vi "plot_side_cutting_offset.vi"(10 "index":dbl, 11 "coord cluster":cluster{dbl[][]}[](array[cluster])) -> (2 "End Point out":cluster{"X":i32, "Y":i32}, 3 "Start Point out":cluster{"X":i32, "Y":i32})   [LabVIEW 2017]
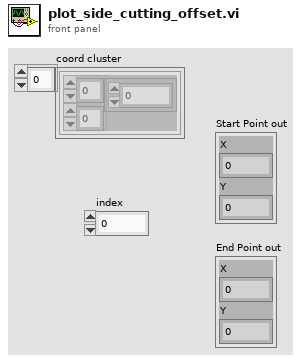
[diagram p1: front panel]
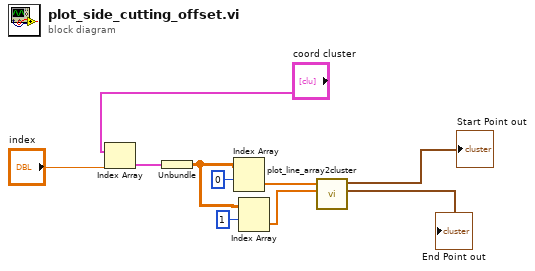
[diagram p0: block diagram]
diagram:
  n1 = Index Array(array="coord cluster", index="index") -> (element=w4:cluster{dbl[][]})
  n2 = Unbundle(w4) -> (w9:dbl[][])
  n3 = Index Array(array=w9, index (row)=0) -> (element=w7:dbl[])  [unwired: 1 in]
  n4 = Index Array(array=w9, index (row)=1) -> (element=w10:dbl[])  [unwired: 1 in]
  n5 = call "plot_line_array2cluster.vi"("End Point array"=w10, "Start Point array"=w7) -> ("End Point out"=→"End Point out":cluster{"X":i32, "Y":i32}, "Start Point out"=→"Start Point out":cluster{"X":i32, "Y":i32})  [unwired: 8 in]
